vi "Close.vi"(8 "error in":errorcluster, 11 "Font in":refnum<class "Font.lvclass">) -> (0 "error out":errorcluster, 3 "Font out":refnum<class "Font.lvclass">)   [LabVIEW 2024, in "Font.lvclass"]
uses:
  Font.lvclass
  Font.lvclass/Font.ctl
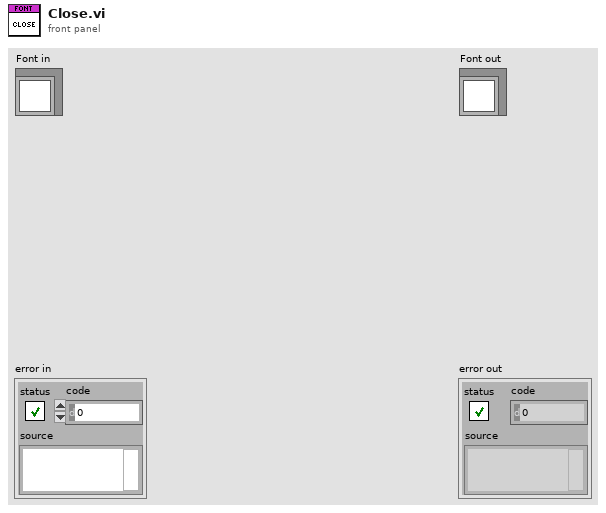
[diagram p1: front panel]
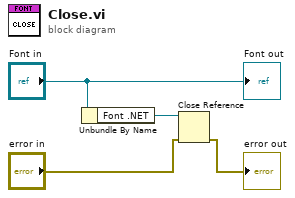
[diagram p0: block diagram]
diagram:
  n1 = Unbundle By Name("Font in") -> ("Font .NET"=w3:refnum<k24>)
  n2 = Close Reference(reference=w3, error in (no error)="error in") -> (error out=→"error out":errorcluster)
  "Font out" <- "Font in"
